vi "Keyence Height Measurement.vi"() -> ()   [LabVIEW 2016]
uses:
  <vilib>/Platform/TimedLoop/XDataNode/timing_clust.ctl
  <vilib>/Platform/TimedLoop/XDataNode/nitl_modes.ctl
  <vilib>/Platform/TimedLoop/XDataNode/wakeup.ctl
  <vilib>/DAQmx/read.llb/DAQmx Read (Digital 1D Bool 1Chan 1Samp).vi
  <vilib>/DAQmx/write.llb/DAQmx Write (Digital Bool 1Line 1Point).vi
  <vilib>/DAQmx/read.llb/DAQmx Read (Analog DBL 1Chan 1Samp).vi
  <vilib>/DAQmx/miscellaneous.llb/DAQmx Fill In Error Info.vi
  <vilib>/Utility/file.llb/Write Delimited Spreadsheet (DBL).vi
  <vilib>/platform/TimedLoop/XDataNode/XDataNode.xnode
  <vilib>/Platform/TimedLoop/XDataNode/XDNodeRunTimeDep.lvlib
panel:
  in  "mm/Volt":dbl=6.0
  in  "Write To File?":bool=TRUE
  out "Ready to Scan":bool
  in  "Keyence On/Open":bool
  out "Waveform Graph":waveform(dbl)(graph)={"t0"=timestamp(0 s since 1904-01-01), "dt"=1.0, "Y"=array[201 elements]}
  in  "Robot Speed":dbl=100.0
  out "Position":dbl=200.0
  out "Height":dbl=-11.328070163726807 format="%0.2f"
  out "Robot Trigger":bool
  in  "stop":bool
  # "mm/s"
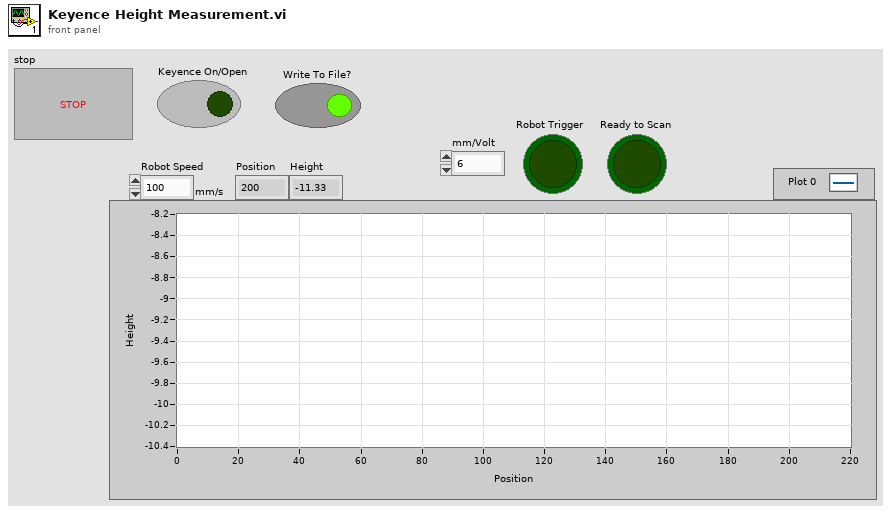
[diagram p1: front panel]
types:
  T1 = typedef "XDNodeRunTimeDep.lvlib/timing_clust.ctl" = cluster{"Expected End [f-1]":u64, "Actual End [f-1]":u64, "Finished Late? [f-1]":bool, "Expected End [i-1]":u64, "Actual End [i-1]":u64, "Finished Late? [i-1]":bool, "Expected Start [i]":u64, "Actual Start [i]":u64, "Expected Start [f]":u64, "Actual Start [f]":u64, "Source Name":string, "Structure Name":string, "Period":i64, "Deadline":i64, "Offset":i64, "Start":i64, "Priority":i32, "Timeout":i32, "Mode":T2, "Wakeup Reason":T3, "Error":errorcluster, "Source Type":string, "Secondary Source Type":string, "Global End Time":u64, "Global Start Time":u64, "Frame Duration":u64, "Iteration Duration":u64, "Assigned CPU":i32, "I/O Scan Engine Mode":u32}
  T2 = typedef "XDNodeRunTimeDep.lvlib/nitl_modes.ctl" = enum32{"No Change", "Process missed periods, maintain original phase", "Discard missed periods, maintain original phase", "Process missed periods, ignore original phase", "Discard missed periods, ignore original phase"}
  T3 = typedef "XDNodeRunTimeDep.lvlib/wakeup.ctl" = enum32{"Normal", "Aborted", "Asynchronous wakeup", "Timing source error", "Timed loop error", "Timeout"}
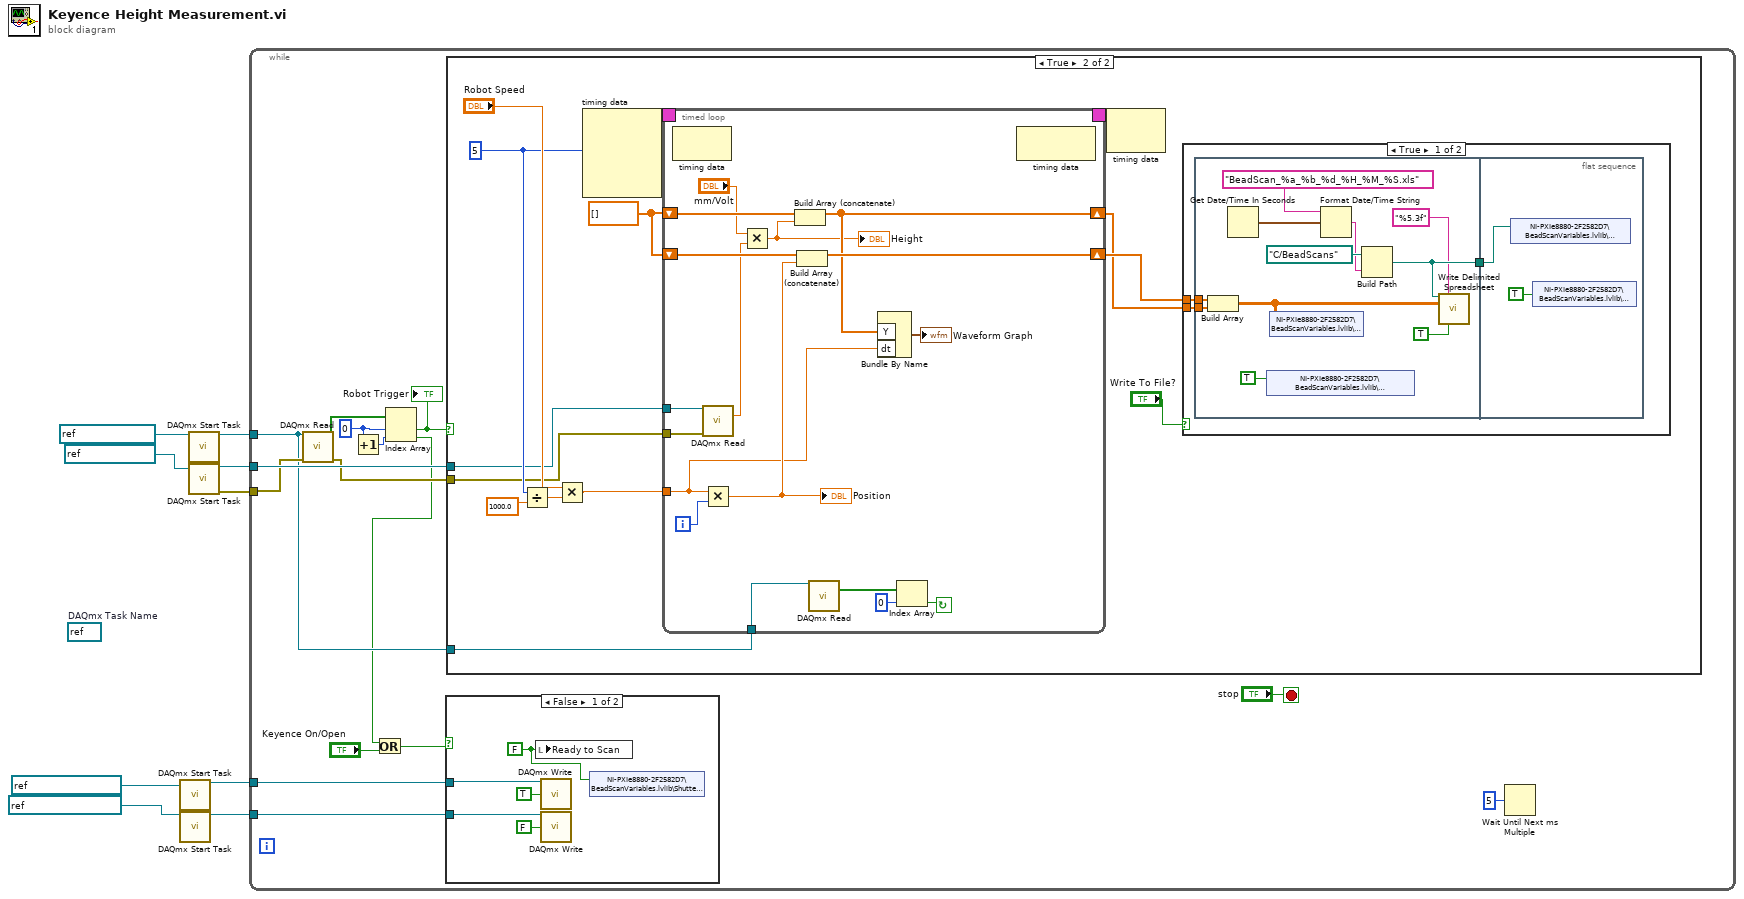
[diagram p0: block diagram]
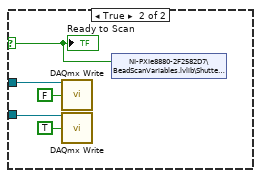
[diagram p2: hidden frame]
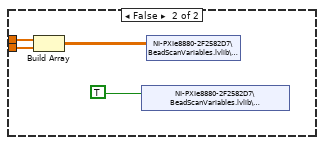
[diagram p4: hidden frame]
diagram:
  (unwired) refnum<k21> refnum  # DAQmx Task Name
  n1 = call <vilib>:"DAQmx Start Task.vi"("task/channels in"=refnum<k21> "Keyence Enable" ("DAQmx Task Name")) -> ("task out"=w1:refnum<k21>, "error out"=w5:errorcluster)  [unwired: 13 in]
  n2 = call <vilib>:"DAQmx Start Task.vi"("task/channels in"=refnum<k21> "Keyence Shutter" ("DAQmx Task Name"), "error in"=w5) -> ("task out"=w2:refnum<k21>)  [unwired: 12 in, 1 out]
  n3 = call <vilib>:"DAQmx Start Task.vi"("task/channels in"=refnum<k21> "Robot Inputs" ("DAQmx Task Name")) -> ("task out"=w10:refnum<k21>, "error out"=w7:errorcluster)  [unwired: 13 in]
  n4 = call <vilib>:"DAQmx Start Task.vi"("task/channels in"=refnum<k21> "Keyence BH" ("DAQmx Task Name"), "error in"=w7) -> ("task out"=w8:refnum<k21>, "error out"=w6:errorcluster)  [unwired: 12 in]
  n5 = while {
    tunnel: w10 -> [w19]
    tunnel: w8 -> [w22]
    tunnel: w6 -> [w20]
    tunnel: w2 -> [w12]
    tunnel: w1 -> [w13]
    stop <- "stop" stop-if-true
    w17 = 0 ("index")
    n6 = call-poly <vilib>:"DAQmx Read.vi"("task/channels in"=w19, "error in"=w20) -> ("data"=w24:bool[], "error out"=w21:errorcluster)  [unwired: 11 in, 1 out]
    n7 = Increment(x=w17) -> (x+1=w18:i32)
    n8 = Index Array(array=w24, index #1=w17, index #2=w18) -> (element #1=w23:bool, element #2=w16:bool)
    "Robot Trigger" <- w23
    n9 = Or(x=w16, y="Keyence On/Open") -> (x .or. y?=w15:bool)
    n10 = case shown="False" w15 {
      selector: w15 -> [_ w32]
      tunnel: w13 -> [w29 w36]
      tunnel: w12 -> [w28 w35]
      frame False {
        w27 = FALSE
        n11 = local write "Ready to Scan"(w27) -> ()
        n12 = call-poly <vilib>:"DAQmx Write.vi"("task/channels in"=w29, "data"=TRUE) -> ()  [unwired: 11 in, 3 out]
        n13 = call-poly <vilib>:"DAQmx Write.vi"("task/channels in"=w28, "data"=FALSE) -> ()  [unwired: 11 in, 3 out]
        n14 = shared-variable "NI-PXIe8880-2F2582D7\\BeadScanVariables.lvlib\\Shutter Open"(w27) -> ()  [unwired: 1 in, 1 out]
      }
      frame True {
        n15 = call-poly <vilib>:"DAQmx Write.vi"("task/channels in"=w36, "data"=FALSE) -> ()  [unwired: 11 in, 3 out]
        n16 = call-poly <vilib>:"DAQmx Write.vi"("task/channels in"=w35, "data"=TRUE) -> ()  [unwired: 11 in, 3 out]
        n17 = shared-variable "NI-PXIe8880-2F2582D7\\BeadScanVariables.lvlib\\Shutter Open"(w32) -> ()  [unwired: 1 in, 1 out]
        "Ready to Scan" <- w32
      }
    }
    n18 = case shown="True" w23 {
      tunnel: w22 -> [_ w43]
      tunnel: w21 -> [_ w42]
      tunnel: w19 -> [_ w41]
      frame False {
      }
      frame True {
        w40 = dbl[] [] ("appended array")
        w45 = i64 5 ("Period")
        n19 = Divide(x=w45, y=1000.0) -> (x/y=w47:dbl)
        n20 = Multiply(x="Robot Speed", y=w47) -> (x*y=w44:dbl)
        n21 = node-c288(w45) -> (w50:T1)  [unwired: 3 in]
        n22 = timed-loop {
          timing: w50 -> [_]
          timing-out: [_] -> w49
          tunnel: w44 -> [w75]
          tunnel: w43 -> [w86]
          tunnel: w42 -> [w85]
          tunnel: w41 -> [w84]
          shift-right: [w76] -> w38
          shift-left: w40 -> [w80]
          shift-right: [w77] -> w39
          shift-left: w40 -> [w78]
          i -> [w87]
          stop <- w81 continue-if-true
          n23 = node-c288() -> ()  [unwired: 1 in, 1 out]
          n24 = call-poly <vilib>:"DAQmx Read.vi"("task/channels in"=w86, "error in"=w85) -> ("data"=w72:dbl)  [unwired: 11 in, 2 out]
          n25 = Multiply(x=w75, y=w87) -> (x*y=w79:dbl)
          "Position" <- w79
          n26 = Multiply(x="mm/Volt", y=w72) -> (x*y=w73:dbl)
          "Height" <- w73
          n27 = Build Array (concatenate)(w80, w73) -> (w76:dbl[])
          n28 = Build Array (concatenate)(w78, w79) -> (w77:dbl[])
          n29 = call-poly <vilib>:"DAQmx Read.vi"("task/channels in"=w84) -> ("data"=w82:bool[])  [unwired: 12 in, 2 out]
          n30 = Bundle By Name("Y"=w76, "dt"=w75) -> (→"Waveform Graph":waveform(dbl))  [unwired: 1 in]
          n31 = Index Array(array=w82, index=0) -> (element=w81:bool)
          n32 = node-c288() -> ()  [unwired: 1 in, 1 out]
        }
        n33 = node-c288(w49) -> ()  [unwired: 1 out]
        n34 = case shown="True" "Write To File?" {
          tunnel: w39 -> [w53 w70]
          tunnel: w38 -> [w52 w69]
          frame True {
            n35 = flat-sequence {
              tunnel: w53 -> [w56]
              tunnel: w52 -> [w55]
              tunnel: [w60] -> w51
              tunnel: w51 -> [w66]
              frame #0 {
                n36 = Build Array(w56, w55) -> (w59:dbl[][])
                n37 = Get Date/Time In Seconds() -> (seconds since 1Jan1904=w63:timestamp)
                n38 = shared-variable "NI-PXIe8880-2F2582D7\\BeadScanVariables.lvlib\\BeadScanComplete"(TRUE ("transpose? (no:F)")) -> ()  [unwired: 1 in, 1 out]
                n39 = shared-variable "NI-PXIe8880-2F2582D7\\BeadScanVariables.lvlib\\ScanData"(w59) -> ()  [unwired: 1 in, 1 out]
                n40 = Format Date/Time String(time format string (%c)="BeadScan_%a_%b_%d_%H_%M_%S.xls", seconds (now)=w63) -> (date/time string=w61:string)  [unwired: 1 in]
                n41 = Build Path(base path=path "C:/BeadScans", name or relative path=w61) -> (appended path=w60:path)
                n42 = call-poly <vilib>:"Write Delimited Spreadsheet.vi"("file path (dialog if empty)"=w60, "format (%.3f)"="%5.3f", "2D data"=w59, "transpose? (no:F)"=TRUE) -> ()  [unwired: 10 in, 2 out]
              }
              frame #1 {
                n43 = shared-variable "NI-PXIe8880-2F2582D7\\BeadScanVariables.lvlib\\BeadScanPath"(w66) -> ()  [unwired: 1 in, 1 out]
                n44 = shared-variable "NI-PXIe8880-2F2582D7\\BeadScanVariables.lvlib\\FileWaiting"(TRUE) -> ()  [unwired: 1 in, 1 out]
              }
            }
          }
          frame False {
            n45 = Build Array(w70, w69) -> (w68:dbl[][])
            n46 = shared-variable "NI-PXIe8880-2F2582D7\\BeadScanVariables.lvlib\\BeadScanComplete"(TRUE) -> ()  [unwired: 1 in, 1 out]
            n47 = shared-variable "NI-PXIe8880-2F2582D7\\BeadScanVariables.lvlib\\ScanData"(w68) -> ()  [unwired: 1 in, 1 out]
          }
        }
      }
    }
    n48 = Wait Until Next ms Multiple(millisecond multiple=u32 5) -> ()  [unwired: 1 out]
  }
